vi "Init SerialIO.vi"(8 "error in":errorcluster, 11 "CRDS in":refnum<class "CRDS.lvclass">=refnum) -> (0 "error out":errorcluster, 2 "SerialCfgOut":cluster{"Q0":dbl[], "T0":sgl}, 3 "CRDS out":refnum<class "CRDS.lvclass">)   [LabVIEW 2012, in "CRDS.lvclass"]
uses:
  CRDS.lvclass
  Reusable/Serial IO/Alicat/AlicatCommBank/AlicatCommBank.lvclass
  Reusable/Serial IO/TE Cooler/TE Cooler.lvclass
  Reusable/Serial IO/Alicat/MC/Alicat_MC.lvclass
  Reusable/TEC/Configuration/TEC Config.ctl
  Devices/Alicat/AlicatCommBank/AlicatCommBank.lvclass
  Devices/Alicat/Alicat.lvclass
  Serial IO/Serial IO.lvclass
  Devices/TE Cooler/TE Cooler.lvclass
  Reusable/DataClass/Alicat/MC/AlicatMCData.lvclass
  Data/Main/CRDS Data.lvclass
  Reusable/DataClass/TECooler/TECData.lvclass
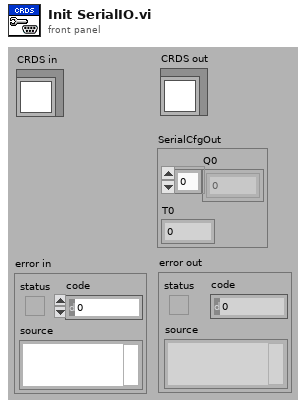
[diagram p1: front panel]
types:
  T1 = cluster{"Address":string[], "Full Scale":dbl[], "Q0":dbl[], "Gas":enum16{"Air", "Ar", "CH4", "CO", "CO2", "C2H6", "H2", "He", "N2", "NO", "Ne", "O2", "C3H8", "n-C4H10", "C2H2", "C2H4", "i-C2H10", "Kr", "Xe"}[], "Port":refnum<visa-resource-name>, "Active":bool[], "Name":string[]}
  T2 = typedef "TEC Config.ctl" = cluster{"T0":sgl, "P":sgl, "I":sgl, "htx":sgl, "D":sgl, "clx":sgl, "Port":refnum<visa-resource-name>, "Active?":bool}
  T3 = typedef "NI_LVConfig.lvlib/Config Data RefNum.ctl" = refnum<k1>
  T4 = enum16{"Air", "Ar", "CH4", "CO", "CO2", "C2H6", "H2", "He", "N2", "NO", "Ne", "O2", "C3H8", "n-C4H10", "C2H2", "C2H4", "i-C2H10", "Kr", "Xe"}[]
  T5 = cluster{"mfcDescr":string, "String":string, "Numeric":dbl, "Gas":enum16{"Air", "Ar", "CH4", "CO", "CO2", "C2H6", "H2", "He", "N2", "NO", "Ne", "O2", "C3H8", "n-C4H10", "C2H2", "C2H4", "i-C2H10", "Kr", "Xe"}}
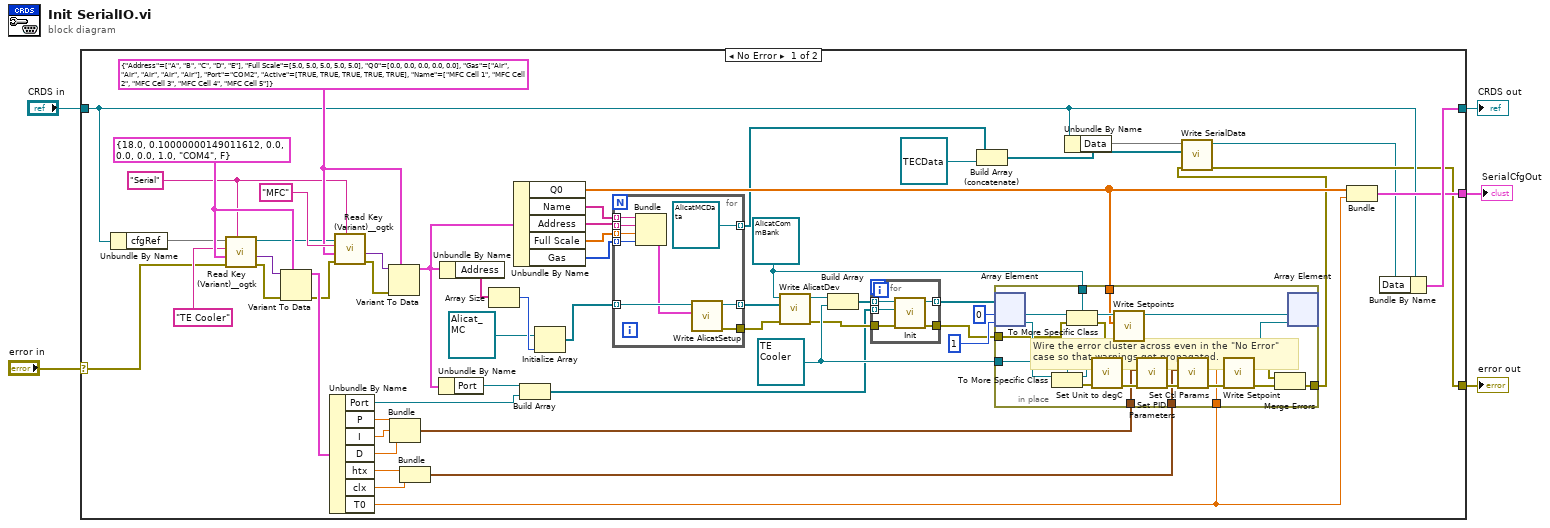
[diagram p0: block diagram]
diagram:
  n1 = case shown="No Error" "error in" {
    selector: "error in" -> [w16 w101]
    tunnel: [w7 w101] -> w4
    tunnel: [w15 w100] -> w2
    tunnel: "CRDS in" -> [w12 w100]
    tunnel: [w14 _] -> w1
    frame No Error {
      w49 = refnum<class "AlicatCommBank.lvclass"> refnum ("AlicatCommBank.lvclass")
      w47 = refnum<class "TE Cooler.lvclass"> refnum ("TE Cooler.lvclass")
      w27 = T1 {"Address"=["A", "B", "C", "D", "E"], "Full Scale"=[5.0, 5.0, 5.0, 5.0, 5.0], "Q0"=[0.0, 0.0, 0.0, 0.0, 0.0], "Gas"=[enum."Air", enum."Air", enum."Air", enum."Air", enum."Air"], "Port"="COM2", "Active"=[TRUE, TRUE, TRUE, TRUE, TRUE], "Name"=["MFC Cell 1", "MFC Cell 2", "MFC Cell 3", "MFC Cell 4", "MFC Cell 5"]} ("flowCfg")
      w23 = T2 {"T0"=18.0, "P"=0.1, "I"=0.0, "htx"=0.0, "D"=0.0, "clx"=1.0, "Port"="COM4", "Active?"=FALSE} ("TEcooler")
      w22 = "Serial" ("section")
      # "Wire the error cluster across even in the \"No Error\"\ncase so that warnings get propagated."
      n2 = Unbundle By Name(w12) -> ("cfgRef"=w17)
      n3 = call <userlib>:"Read Key (Variant)__ogtk.vi"("section"=w22, "error in (no error)"=w16, "type"=w23, "key (optional)"="TE Cooler", "refnum"=w17) -> ("error out"=w19:errorcluster, "key-value"=w20:variant, "refnum out"=w21:T3)  [unwired: 3 in, 1 out]
      n4 = Variant To Data(error in=w19, type=w23, Variant=w20) -> (data=w38:T2, error out=w24:errorcluster)
      n5 = Unbundle By Name(w38) -> ("Port"=w41:refnum<visa-resource-name>, "P"=w50:sgl, "I"=w51:sgl, "D"=w52:sgl, "htx"=w53:sgl, "clx"=w54:sgl, "T0"=w61:sgl)
      n6 = call <userlib>:"Read Key (Variant)__ogtk.vi"("section"=w22, "error in (no error)"=w24, "type"=w27, "key (optional)"="MFC", "refnum"=w21) -> ("error out"=w25:errorcluster, "key-value"=w26:variant)  [unwired: 3 in, 2 out]
      n7 = Variant To Data(error in=w25, type=w27, Variant=w26) -> (data=w39:T1)  [unwired: 1 out]
      n8 = Bundle("P"=w50, "I"=w51, "D"=w52) -> (w56:cluster{"P":sgl, "I":sgl, "D":sgl})  [unwired: 1 in]
      n9 = Bundle("htx"=w53, "clx"=w54) -> (w55:cluster{"htx":sgl, "clx":sgl})  [unwired: 1 in]
      n10 = Unbundle By Name(w39) -> ("Port"=w40:refnum<visa-resource-name>)
      n11 = Unbundle By Name(w39) -> ("Address"=w29:string[])
      n12 = Array Size(array=w29) -> (size(s)=w30:i32)
      n13 = Unbundle By Name(w39) -> ("Q0"=w60:dbl[], "Name"=w37:string[], "Address"=w33:string[], "Full Scale"=w32:dbl[], "Gas"=w34:T4)
      n14 = Build Array(w40, w41) -> (w44:refnum<visa-resource-name>[])
      n15 = Initialize Array(refnum<class "Alicat_MC.lvclass"> refnum ("Alicat_MC.lvclass"), w30) -> (w31:refnum<class "Alicat_MC.lvclass">[])
      n16 = for {
        tunnel: w31 -> [w99] mode=indexing
        tunnel: w32 -> [w97] mode=indexing
        tunnel: w33 -> [w98] mode=indexing
        tunnel: w34 -> [w96] mode=indexing
        tunnel: [w94] -> w35
        tunnel: [w93] -> w36 mode=indexing
        tunnel: w37 -> [w92] mode=indexing
        tunnel: [refnum<class "AlicatMCData.lvclass"> refnum ("AlicatMCData.lvclass")] -> w13 mode=indexing
        n17 = Bundle("mfcDescr"=w92, "String"=w98, "Numeric"=w97, "Gas"=w96) -> (w95:T5)  [unwired: 1 in]
        n18 = call "Write AlicatSetup.vi"("AlicatSetup"=w95, "Alicat in"=w99) -> ("error out"=w94:errorcluster, "Alicat out"=w93:refnum<class "Alicat.lvclass">)  [unwired: 8 in]
      }
      n19 = call "Write AlicatDev.vi"("error in"=w35, "AlicatDev"=w36, "AlicatCommBank in"=w49) -> ("error out"=w45:errorcluster, "AlicatCommBank out"=w42:refnum<class "AlicatCommBank.lvclass">)  [unwired: 7 in]
      n20 = Build Array(w42, w47) -> (w43:refnum<class>[])
      n21 = for {
        tunnel: w43 -> [w90] mode=indexing
        tunnel: w44 -> [w89] mode=indexing
        tunnel: w45 -> [w88]
        tunnel: [w87] -> w46 mode=indexing
        tunnel: [w86] -> w48
        n22 = call-dynamic "Init.vi"("error in"=w88, "Port"=w89, "Serial IO in"=w90) -> ("error out"=w86:errorcluster, "Serial IO out"=w87:refnum<class "Serial IO.lvclass">)  [unwired: 7 in]
      }
      n23 = Build Array (concatenate)(w13, refnum<class "TECData.lvclass"> refnum ("TECData.lvclass")) -> (w9:refnum<class>[])
      n24 = in-place {
        in-place-border: w47 -> [w84]
        in-place-border: w48 -> [w69]
        in-place-border: w49 -> [w77]
        in-place-border: [w66] -> w8
        in-place-border: w55 -> [w65]
        in-place-border: w56 -> [w64]
        in-place-border: w61 -> [w63]
        in-place-border: w60 -> [w62]
        n25 = in-place-array #1(w46, 0, 1) -> (w78:refnum<class "Serial IO.lvclass">, w85:refnum<class "Serial IO.lvclass">)
        n26 = To More Specific Class(target class=w84, reference=w85) -> (specific class reference=w74:refnum<class "TE Cooler.lvclass">, error out=w73:errorcluster)  [unwired: 1 in]
        n27 = To More Specific Class(target class=w77, reference=w78, error in=w69) -> (specific class reference=w76:refnum<class "AlicatCommBank.lvclass">, error out=w70:errorcluster)
        n28 = call "Set Unit to degC.vi"("error in"=w73, "TE Cooler in"=w74) -> ("error out"=w71:errorcluster, "TE Cooler out"=w72:refnum<class "TE Cooler.lvclass">)  [unwired: 8 in]
        n29 = call-dynamic "Write Setpoints.vi"("error in"=w70, "Setpoints"=w62, "AlicatCommBank in"=w76) -> ("error out"=w67:errorcluster, "AlicatCommBank out"=w75:refnum<class "AlicatCommBank.lvclass">)  [unwired: 7 in]
        n30 = call "Set PID Parameters.vi"("error in (no error)"=w71, "PID Params"=w64, "TE Cooler in"=w72) -> ("error out"=w82:errorcluster, "TE Cooler out"=w83:refnum<class "TE Cooler.lvclass">)  [unwired: 7 in]
        n31 = call "Set Ctl Params.vi"("error in (no error)"=w82, "Ctl Params"=w65, "TE Cooler in"=w83) -> ("error out"=w80:errorcluster, "TE Cooler out"=w81:refnum<class "TE Cooler.lvclass">)  [unwired: 7 in]
        n32 = call "Write Setpoint.vi"("error in"=w80, "SP"=w63, "TE Cooler in"=w81) -> ("error out"=w68:errorcluster, "TE Cooler out"=w79:refnum<class "TE Cooler.lvclass">)  [unwired: 7 in]
        n33 = Merge Errors(w67, w68) -> (w66:errorcluster)
        n34 = in-place-array #1(w75, w79) -> ()  [unwired: 3 out]
      }
      n35 = Unbundle By Name(w12) -> ("Data"=w11)
      n36 = call "Write SerialData.vi"("error in (no error)"=w8, "SerialData"=w9, "CRDS Data in"=w11) -> ("error out"=w7:errorcluster, "CRDS Data out"=w6:refnum<class "CRDS Data.lvclass">)  [unwired: 7 in]
      n37 = Bundle("Q0"=w60, "T0"=w61) -> (w14:cluster{"Q0":dbl[], "T0":sgl})  [unwired: 1 in]
      n38 = Bundle By Name(cluster=w12, "Data"=w6) -> (w15:cluster{})
    }
    frame Error {
    }
  }
  "error out" <- w4
  "CRDS out" <- w2
  "SerialCfgOut" <- w1
